vi "DatabaseHand_findGroup.vi"(9 "group":string, 10 "Data In":T2) -> (2 "group":T1[](array[typedef]))   [LabVIEW 2016]
uses:
  DatabaseHand_Element.ctl
  DatabaseHan_DatabaseElement.ctl
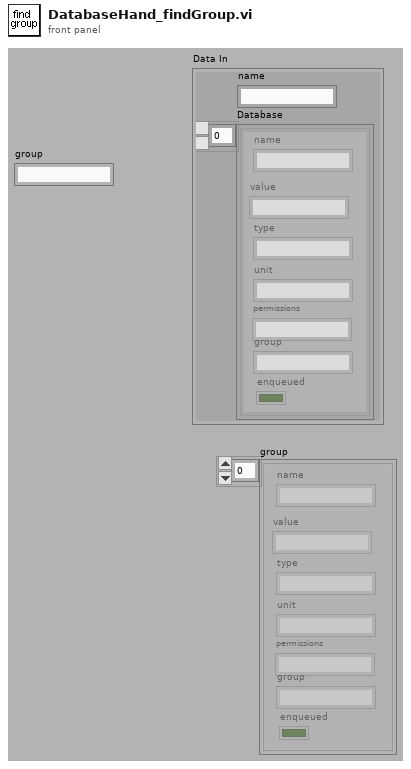
[diagram p1: front panel]
types:
  T1 = typedef "DatabaseHan_DatabaseElement.ctl" = cluster{"name":string, "value":string, "type":string, "unit":string, "permissions":string, "enqueued":bool, "group":string}
  T2 = typedef "DatabaseHand_Element.ctl" = cluster{"name":string, "Database":T1[]}
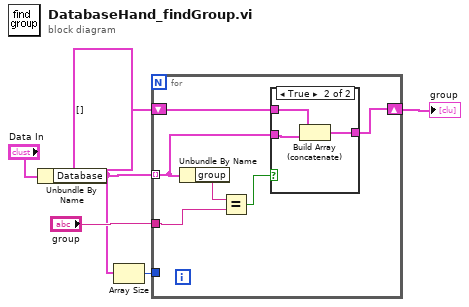
[diagram p0: block diagram]
diagram:
  n1 = Unbundle By Name("Data In") -> ("Database"=w4:T1[])
  n2 = Array Size(array=w4) -> (size(s)=w3:i32)
  n3 = for {
    tunnel: w4 -> [w9] mode=indexing
    tunnel: "group" -> [w11]
    tunnel: w3 -> [_]
    shift-right: [w8] -> w1
    shift-left: T1[] [] -> [w7]
    n4 = Unbundle By Name(w9) -> ("group"=w12:string)
    n5 = Equal?(x=w12, y=w11) -> (x = y?=w10:bool)
    n6 = case shown="True" w10 {
      tunnel: w9 -> [_ w16]
      tunnel: [w13 w15] -> w8
      tunnel: w7 -> [w13 w14]
      frame False {
      }
      frame True {
        n7 = Build Array (concatenate)(w14, w16) -> (w15:T1[])
      }
    }
  }
  "group" <- w1
